vi "Message_Manager.vi"(6 "Log only on Err":bool, 7 "Action (Add)":T1, 8 "error in":errorcluster, 10 "New Entry":string, 11 "Log History Size (1000)":i32=1000) -> (0 "error out":errorcluster, 2 "Last Err":cluster{"code":i32, "source":string}, 3 "First Err (Latched)":cluster{"code":i32, "source":string}, 4 "Last Message":string="12/05/2020 06:01:50.239 PM -- hello world", 5 "Message Log":string="12/05/2020 06:01:50.239 PM -- hello world\r\n12/05/2020 06:01:50.238 PM -- hello world\r\n12/05/2020 06:01:50.237 PM -- hello world\r\n12/05/2020 06:01:50.237 PM -- hello world\r\n12/05/2020 06:01:50.236 PM -- hello world\r\n12/05/2020 06:01:50.235 PM -- hello world\r\n12/05/2020 06:01:50.234 PM -- hello world\r\n12/05/2020 06:01:50.234 PM -- hello world\r\n12/05/2020 06:01:50.233 PM -- hello world\r\n12/05/2020 06:01:50.232 PM -- hello world\r\n12/05/2020 06:01:50.231 PM -- hello world\r\n12/05/2020 06:01:50.231 PM -- hello world\r\n12/05/2020 06:01:50.230 PM -- hello world\r\n12/05/2020 06:01:50.227 PM -- hello world\r\n12/05/2020 06:01:50.227 PM -- hello world\r\n12/05/2020 06:01:50.226 PM -- hello world\r\n12/05/2020 06:01:50.225 PM -- hello world\r\n12/05/2020 06:01:50.224 PM -- hello world\r\n12/05/2020 06:01:50.224 PM -- hello world\r\n12/05/2020 06:01:50.223 PM -- hello world\r\n12/05/2020 06:01:50.222 PM -- hello world\r\n12/05/2020 06:01:50.221 PM -- hello world\r\n12/05/2020 06:01:50.221 PM -- hello world\r\n12/05/2020 06:01:50.220 PM -- hello world\r\n12/05/2020 06:01:50.219 PM -- hello world\r\n12/05/2020 06:01:50.218 PM -- hello world\r\n12/05/2020 06:01:50.218 PM -- hello world\r\n12/05/2020 06:01:50.217 PM -- hello world\r\n12/05/2020 06:01:50.216 PM -- hello world\r\n12/05/2020 06:01:50.215 PM -- hello world\r\n12/05/2020 06:01:50.215 PM -- hello world\r\n12/05/2020 06:01:50.215 PM -- hello world\r\n12/05/2020 06:01:50.213 PM -- hello world\r\n12/05/2020 06:01:50.211 PM -- hello world\r\n12/05/2020 06:01:50.211 PM -- hello world\r\n12/05/2020 06:01:50.210 PM -- hello world\r\n12/05/2020 06:01:50.209 PM -- hello world\r\n12/05/2020 06:01:50.208 PM -- hello world\r\n12/05/2020 06:01:50.208 PM -- hello world\r\n12/05/2020 06:01:50.207 PM -- hello world\r\n12/05/2020 06:01:50.206 PM -- hello world\r\n12/05/2020 06:01:50.205 PM -- hello world\r\n12/05/2020 06:01:50.205 PM -- hello world\r\n12/05/2020 06:01:50.204 PM -- hello world\r\n12/05/2020 06:01:50.203 PM -- hello world\r\n12/05/2020 06:01:50.203 PM -- hello world\r\n12/05/2020 06:01:50.202 PM -- hello world\r\n12/05/2020 06:01:50.201 PM -- hello world\r\n12/05/2020 06:01:50.200 PM -- hello world\r\n12/05/2020 06:01:50.200 PM -- hello world\r\n12/05/2020 06:01:50.199 PM -- hello world\r\n12/05/2020 06:01:50.198 PM -- hello world\r\n12/05/2020 06:01:50.196 PM -- hello world\r\n12/05/2020 06:01:50.195 PM -- hello world\r\n12/05/2020 06:01:50.194 PM -- hello world\r\n12/05/2020 06:01:50.193 PM -- hello world\r\n12/05/2020 06:01:50.193 PM -- hello world\r\n12/05/2020 06:01:50.192 PM -- hello world\r\n12/05/2020 06:01:50.191 PM -- hello world\r\n12/05/2020 06:01:50.191 PM -- hello world\r\n12/05/2020 06:01:50.190 PM -- hello world\r\n12/05/2020 06:01:50.189 PM -- hello world\r\n12/05/2020 06:01:50.188 PM -- hello world\r\n12/05/2020 06:01:50.188 PM -- hello world\r\n12/05/2020 06:01:50.187 PM -- hello world\r\n12/05/2020 06:01:50.186 PM -- hello world\r\n12/05/2020 06:01:50.186 PM -- hello world\r\n12/05/2020 06:01:50.185 PM -- hello world\r\n12/05/2020 06:01:50.184 PM -- hello world\r\n12/05/2020 06:01:50.183 PM -- hello world\r\n12/05/2020 06:01:50.182 PM -- hello world\r\n12/05/2020 06:01:50.180 PM -- hello world\r\n12/05/2020 06:01:50.179 PM -- hello world\r\n12/05/2020 06:01:50.179 PM -- hello world\r\n12/05/2020 06:01:50.178 PM -- hello world\r\n12/05/2020 06:01:50.177 PM -- hello world\r\n12/05/2020 06:01:50.176 PM -- hello world\r\n12/05/2020 06:01:50.175 PM -- hello world\r\n12/05/2020 06:01:50.175 PM -- hello world\r\n12/05/2020 06:01:50.174 PM -- hello world\r\n12/05/2020 06:01:50.173 PM -- hello world\r\n12/05/2020 06:01:50.173 PM -- hello world\r\n12/05/2020 06:01:50.173 PM -- hello world\r\n12/05/2020 06:01:50.172 PM -- hello world\r\n12/05/2020 06:01:50.171 PM -- hello world\r\n12/05/2020 06:01:50.171 PM -- hello world\r\n12/05/2020 06:01:50.170 PM -- hello world\r\n12/05/2020 06:01:50.169 PM -- hello world\r\n12/05/2020 06:01:50.168 PM -- hello world\r\n12/05/2020 06:01:50.167 PM -- hello world\r\n12/05/2020 06:01:50.166 PM -- hello world\r\n12/05/2020 06:01:50.166 PM -- hello world\r\n12/05/2020 06:01:50.165 PM -- hello world\r\n12/05/2020 06:01:50.164 PM -- hello world\r\n12/05/2020 06:01:50.164 PM -- hello world\r\n12/05/2020 06:01:50.163 PM -- hello world\r\n12/05/2020 06:01:50.161 PM -- hello world\r\n12/05/2020 06:01:50.160 PM -- hello world\r\n12/05/2020 06:01:50.159 PM -- hello world\r\n12/05/2020 06:01:50.159 PM -- hello world\r\n12/05/2020 06:01:50.158 PM -- hello world\r\n12/05/2020 06:01:50.157 PM -- hello world\r\n12/05/2020 06:01:50.156 PM -- hello world\r\n12/05/2020 06:01:50.156 PM -- hello world\r\n12/05/2020 06:01:50.155 PM -- hello world\r\n12/05/2020 06:01:50.154 PM -- hello world\r\n12/05/2020 06:01:50.153 PM -- hello world\r\n12/05/2020 06:01:50.153 PM -- hello world\r\n12/05/2020 06:01:50.152 PM -- hello world\r\n12/05/2020 06:01:50.151 PM -- hello world\r\n12/05/2020 06:01:50.150 PM -- hello world\r\n12/05/2020 06:01:50.148 PM -- hello world\r\n12/05/2020 06:01:50.147 PM -- hello world\r\n12/05/2020 06:01:50.147 PM -- hello world\r\n12/05/2020 06:01:50.146 PM -- hello world\r\n12/05/2020 06:01:50.145 PM -- hello world\r\n12/05/2020 06:01:50.144 PM -- hello world\r\n12/05/2020 06:01:50.143 PM -- hello world\r\n12/05/2020 06:01:50.142 PM -- hello world\r\n12/05/2020 06:01:50.142 PM -- hello world\r\n12/05/2020 06:01:50.141 PM -- hello world\r\n12/05/2020 06:01:50.140 PM -- hello world\r\n12/05/2020 06:01:50.139 PM -- hello world\r\n12/05/2020 06:01:50.138 PM -- hello world\r\n12/05/2020 06:01:50.137 PM -- hello world\r\n12/05/2020 06:01:50.137 PM -- hello world\r\n12/05/2020 06:01:50.136 PM -- hello world\r\n12/05/2020 06:01:50.135 PM -- hello world\r\n12/05/2020 06:01:50.133 PM -- hello world\r\n12/05/2020 06:01:50.133 PM -- hello world\r\n12/05/2020 06:01:50.132 PM -- hello world\r\n12/05/2020 06:01:50.131 PM -- hello world\r\n12/05/2020 06:01:50.130 PM -- hello world\r\n12/05/2020 06:01:50.130 PM -- hello world\r\n12/05/2020 06:01:50.130 PM -- hello world\r\n12/05/2020 06:01:50.129 PM -- hello world\r\n12/05/2020 06:01:50.128 PM -- hello world\r\n12/05/2020 06:01:50.127 PM -- hello world\r\n12/05/2020 06:01:50.127 PM -- hello world\r\n12/05/2020 06:01:50.126 PM -- hello world\r\n12/05/2020 06:01:50.125 PM -- hello world\r\n12/05/2020 06:01:50.124 PM -- hello world\r\n12/05/2020 06:01:50.124 PM -- hello world\r\n12/05/2020 06:01:50.123 PM -- hello world\r\n12/05/2020 06:01:50.122 PM -- hello world\r\n12/05/2020 06:01:50.121 PM -- hello world\r\n12/05/2020 06:01:50.121 PM -- hello world\r\n12/05/2020 06:01:50.120 PM -- hello world\r\n12/05/2020 06:01:50.119 PM -- hello world\r\n12/05/2020 06:01:50.118 PM -- hello world\r\n12/05/2020 06:01:50.117 PM -- hello world\r\n12/05/2020 06:01:50.117 PM -- hello world\r\n12/05/2020 06:01:50.116 PM -- hello world\r\n12/05/2020 06:01:50.115 PM -- hello world\r\n12/05/2020 06:01:50.114 PM -- hello world\r\n12/05/2020 06:01:50.114 PM -- hello world\r\n12/05/2020 06:01:50.113 PM -- hello world\r\n12/05/2020 06:01:50.112 PM -- hello world\r\n12/05/2020 06:01:50.111 PM -- hello world\r\n12/05/2020 06:01:50.111 PM -- hello world\r\n12/05/2020 06:01:50.110 PM -- hello world\r\n12/05/2020 06:01:50.109 PM -- hello world\r\n12/05/2020 06:01:50.108 PM -- hello world\r\n12/05/2020 06:01:50.108 PM -- hello world\r\n12/05/2020 06:01:50.107 PM -- hello world\r\n12/05/2020 06:01:50.106 PM -- hello world\r\n12/05/2020 06:01:50.105 PM -- hello world\r\n12/05/2020 06:01:50.105 PM -- hello world\r\n12/05/2020 06:01:50.102 PM -- hello world\r\n12/05/2020 06:01:50.102 PM -- hello world\r\n12/05/2020 06:01:50.101 PM -- hello world\r\n12/05/2020 06:01:50.100 PM -- hello world\r\n12/05/2020 06:01:50.099 PM -- hello world\r\n12/05/2020 06:01:50.099 PM -- hello world\r\n12/05/2020 06:01:50.098 PM -- hello world\r\n12/05/2020 06:01:50.097 PM -- hello world\r\n12/05/2020 06:01:50.096 PM -- hello world\r\n12/05/2020 06:01:50.096 PM -- hello world\r\n12/05/2020 06:01:50.095 PM -- hello world\r\n12/05/2020 06:01:50.094 PM -- hello world\r\n12/05/2020 06:01:50.093 PM -- hello world\r\n12/05/2020 06:01:50.092 PM -- hello world\r\n12/05/2020 06:01:50.091 PM -- hello world\r\n12/05/2020 06:01:50.091 PM -- hello world\r\n12/05/2020 06:01:50.090 PM -- hello world\r\n12/05/2020 06:01:50.090 PM -- hello world\r\n12/05/2020 06:01:50.090 PM -- hello world\r\n12/05/2020 06:01:50.089 PM -- hello world\r\n12/05/2020 06:01:50.086 PM -- hello world\r\n12/05/2020 06:01:50.086 PM -- hello world\r\n12/05/2020 06:01:50.085 PM -- hello world\r\n12/05/2020 06:01:50.084 PM -- hello world\r\n12/05/2020 06:01:50.083 PM -- hello world\r\n12/05/2020 06:01:50.083 PM -- hello world\r\n12/05/2020 06:01:50.082 PM -- hello world\r\n12/05/2020 06:01:50.081 PM -- hello world\r\n12/05/2020 06:01:50.080 PM -- hello world\r\n12/05/2020 06:01:50.079 PM -- hello world\r\n12/05/2020 06:01:50.077 PM -- hello world\r\n12/05/2020 06:01:50.075 PM -- hello world\r\n12/05/2020 06:01:50.073 PM -- hello world\r\n12/05/2020 06:01:50.073 PM -- hello world\r\n12/05/2020 06:01:50.072 PM -- hello world\r\n12/05/2020 06:01:50.071 PM -- hello world\r\n12/05/2020 06:01:50.070 PM -- hello world\r\n12/05/2020 06:01:50.070 PM -- hello world\r\n12/05/2020 06:01:50.069 PM -- hello world\r\n12/05/2020 06:01:50.068 PM -- hello world\r\n12/05/2020 06:01:50.067 PM -- hello world\r\n12/05/2020 06:01:50.066 PM -- hello world\r\n12/05/2020 06:01:50.066 PM -- hello world\r\n12/05/2020 06:01:50.065 PM -- hello world\r\n12/05/2020 06:01:50.064 PM -- hello world\r\n12/05/2020 06:01:50.064 PM -- hello world\r\n12/05/2020 06:01:50.063 PM -- hello world\r\n12/05/2020 06:01:50.062 PM -- hello world\r\n12/05/2020 06:01:50.061 PM -- hello world\r\n12/05/2020 06:01:50.060 PM -- hello world\r\n12/05/2020 06:01:50.059 PM -- hello world\r\n12/05/2020 06:01:50.058 PM -- hello world\r\n12/05/2020 06:01:50.056 PM -- hello world\r\n12/05/2020 06:01:50.053 PM -- hello world\r\n12/05/2020 06:01:50.051 PM -- hello world\r\n12/05/2020 06:01:50.049 PM -- hello world\r\n12/05/2020 06:01:50.048 PM -- hello world\r\n12/05/2020 06:01:50.046 PM -- hello world\r\n12/05/2020 06:01:50.042 PM -- hello world\r\n12/05/2020 06:01:50.039 PM -- hello world\r\n12/05/2020 06:01:50.038 PM -- hello world\r\n12/05/2020 06:01:50.037 PM -- hello world\r\n12/05/2020 06:01:50.037 PM -- hello world\r\n12/05/2020 06:01:50.036 PM -- hello world\r\n12/05/2020 06:01:50.035 PM -- hello world\r\n12/05/2020 06:01:50.034 PM -- hello world\r\n12/05/2020 06:01:50.033 PM -- hello world\r\n12/05/2020 06:01:50.033 PM -- hello world\r\n12/05/2020 06:01:50.032 PM -- hello world\r\n12/05/2020 06:01:50.031 PM -- hello world\r\n12/05/2020 06:01:50.031 PM -- hello world\r\n12/05/2020 06:01:50.030 PM -- hello world\r\n12/05/2020 06:01:50.029 PM -- hello world\r\n12/05/2020 06:01:50.028 PM -- hello world\r\n12/05/2020 06:01:50.026 PM -- hello world\r\n12/05/2020 06:01:50.023 PM -- hello world\r\n12/05/2020 06:01:50.023 PM -- hello world\r\n12/05/2020 06:01:50.022 PM -- hello world\r\n12/05/2020 06:01:50.021 PM -- hello world\r\n12/05/2020 06:01:50.020 PM -- hello world\r\n12/05/2020 06:01:50.020 PM -- hello world\r\n12/05/2020 06:01:50.019 PM -- hello world\r\n12/05/2020 06:01:50.018 PM -- hello world\r\n12/05/2020 06:01:50.017 PM -- hello world\r\n12/05/2020 06:01:50.016 PM -- hello world\r\n12/05/2020 06:01:50.015 PM -- hello world\r\n12/05/2020 06:01:50.014 PM -- hello world\r\n12/05/2020 06:01:50.013 PM -- hello world\r\n12/05/2020 06:01:50.012 PM -- hello world\r\n12/05/2020 06:01:50.012 PM -- hello world\r\n12/05/2020 06:01:50.011 PM -- hello world\r\n12/05/2020 06:01:50.010 PM -- hello world\r\n12/05/2020 06:01:50.009 PM -- hello world\r\n12/05/2020 06:01:50.009 PM -- hello world\r\n12/05/2020 06:01:50.007 PM -- hello world\r\n12/05/2020 06:01:50.006 PM -- hello world\r\n12/05/2020 06:01:50.006 PM -- hello world\r\n12/05/2020 06:01:50.006 PM -- hello world\r\n12/05/2020 06:01:50.005 PM -- hello world\r\n12/05/2020 06:01:50.004 PM -- hello world\r\n12/05/2020 06:01:50.004 PM -- hello world\r\n12/05/2020 06:01:50.003 PM -- hello world\r\n12/05/2020 06:01:50.002 PM -- hello world\r\n12/05/2020 06:01:50.001 PM -- hello world\r\n12/05/2020 06:01:50.001 PM -- hello world\r\n12/05/2020 06:01:50.000 PM -- hello world\r\n12/05/2020 06:01:49.999 PM -- hello world\r\n12/05/2020 06:01:49.999 PM -- hello world\r\n12/05/2020 06:01:49.998 PM -- hello world\r\n12/05/2020 06:01:49.997 PM -- hello world\r\n12/05/2020 06:01:49.994 PM -- hello world\r\n12/05/2020 06:01:49.993 PM -- hello world\r\n12/05/2020 06:01:49.992 PM -- hello world\r\n12/05/2020 06:01:49.991 PM -- hello world\r\n12/05/2020 06:01:49.991 PM -- hello world\r\n12/05/2020 06:01:49.990 PM -- hello world\r\n12/05/2020 06:01:49.989 PM -- hello world\r\n12/05/2020 06:01:49.988 PM -- hello world\r\n12/05/2020 06:01:49.988 PM -- hello world\r\n12/05/2020 06:01:49.987 PM -- hello world\r\n12/05/2020 06:01:49.986 PM -- hello world\r\n12/05/2020 06:01:49.986 PM -- hello world\r\n12/05/2020 06:01:49.985 PM -- hello world\r\n12/05/2020 06:01:49.984 PM -- hello world\r\n12/05/2020 06:01:49.983 PM -- hello world\r\n12/05/2020 06:01:49.982 PM -- hello world\r\n12/05/2020 06:01:49.982 PM -- hello world\r\n12/05/2020 06:01:49.981 PM -- hello world\r\n12/05/2020 06:01:49.980 PM -- hello world\r\n12/05/2020 06:01:49.980 PM -- hello world\r\n12/05/2020 06:01:49.979 PM -- hello world\r\n12/05/2020 06:01:49.976 PM -- hello world\r\n12/05/2020 06:01:49.976 PM -- hello world\r\n12/05/2020 06:01:49.975 PM -- hello world\r\n12/05/2020 06:01:49.974 PM -- hello world\r\n12/05/2020 06:01:49.973 PM -- hello world\r\n12/05/2020 06:01:49.973 PM -- hello world\r\n12/05/2020 06:01:49.972 PM -- hello world\r\n12/05/2020 06:01:49.971 PM -- hello world\r\n12/05/2020 06:01:49.971 PM -- hello world\r\n12/05/2020 06:01:49.970 PM -- hello world\r\n12/05/2020 06:01:49.969 PM -- hello world\r\n12/05/2020 06:01:49.968 PM -- hello world\r\n12/05/2020 06:01:49.968 PM -- hello world\r\n12/05/2020 06:01:49.967 PM -- hello world\r\n12/05/2020 06:01:49.966 PM -- hello world\r\n12/05/2020 06:01:49.965 PM -- hello world\r\n12/05/2020 06:01:49.965 PM -- hello world\r\n12/05/2020 06:01:49.965 PM -- hello world\r\n12/05/2020 06:01:49.963 PM -- hello world\r\n12/05/2020 06:01:49.961 PM -- hello world\r\n12/05/2020 06:01:49.960 PM -- hello world\r\n12/05/2020 06:01:49.960 PM -- hello world\r\n12/05/2020 06:01:49.959 PM -- hello world\r\n12/05/2020 06:01:49.958 PM -- hello world\r\n12/05/2020 06:01:49.957 PM -- hello world\r\n12/05/2020 06:01:49.957 PM -- hello world\r\n12/05/2020 06:01:49.956 PM -- hello world\r\n12/05/2020 06:01:49.955 PM -- hello world\r\n12/05/2020 06:01:49.955 PM -- hello world\r\n12/05/2020 06:01:49.954 PM -- hello world\r\n12/05/2020 06:01:49.953 PM -- hello world\r\n12/05/2020 06:01:49.952 PM -- hello world\r\n12/05/2020 06:01:49.952 PM -- hello world\r\n12/05/2020 06:01:49.951 PM -- hello world\r\n12/05/2020 06:01:49.950 PM -- hello world\r\n12/05/2020 06:01:49.949 PM -- hello world\r\n12/05/2020 06:01:49.948 PM -- hello world\r\n12/05/2020 06:01:49.948 PM -- hello world\r\n12/05/2020 06:01:49.945 PM -- hello world\r\n12/05/2020 06:01:49.944 PM -- hello world\r\n12/05/2020 06:01:49.944 PM -- hello world\r\n12/05/2020 06:01:49.942 PM -- hello world\r\n12/05/2020 06:01:49.941 PM -- hello world\r\n12/05/2020 06:01:49.940 PM -- hello world\r\n12/05/2020 06:01:49.940 PM -- hello world\r\n12/05/2020 06:01:49.939 PM -- hello world\r\n12/05/2020 06:01:49.938 PM -- hello world\r\n12/05/2020 06:01:49.938 PM -- hello world\r\n12/05/2020 06:01:49.937 PM -- hello world\r\n12/05/2020 06:01:49.936 PM -- hello world\r\n12/05/2020 06:01:49.935 PM -- hello world\r\n12/05/2020 06:01:49.935 PM -- hello world\r\n12/05/2020 06:01:49.933 PM -- hello world\r\n12/05/2020 06:01:49.932 PM -- hello world\r\n12/05/2020 06:01:49.930 PM -- hello world\r\n12/05/2020 06:01:49.929 PM -- hello world\r\n12/05/2020 06:01:49.928 PM -- hello world\r\n12/05/2020 06:01:49.928 PM -- hello world\r\n12/05/2020 06:01:49.927 PM -- hello world\r\n12/05/2020 06:01:49.926 PM -- hello world\r\n12/05/2020 06:01:49.925 PM -- hello world\r\n12/05/2020 06:01:49.925 PM -- hello world\r\n12/05/2020 06:01:49.924 PM -- hello world\r\n12/05/2020 06:01:49.923 PM -- hello world\r\n12/05/2020 06:01:49.923 PM -- hello world\r\n12/05/2020 06:01:49.923 PM -- hello world\r\n12/05/2020 06:01:49.922 PM -- hello world\r\n12/05/2020 06:01:49.921 PM -- hello world\r\n12/05/2020 06:01:49.921 PM -- hello world\r\n12/05/2020 06:01:49.920 PM -- hello world\r\n12/05/2020 06:01:49.919 PM -- hello world\r\n12/05/2020 06:01:49.919 PM -- hello world\r\n12/05/2020 06:01:49.918 PM -- hello world\r\n12/05/2020 06:01:49.917 PM -- hello world\r\n12/05/2020 06:01:49.916 PM -- hello world\r\n12/05/2020 06:01:49.914 PM -- hello world\r\n12/05/2020 06:01:49.914 PM -- hello world\r\n12/05/2020 06:01:49.913 PM -- hello world\r\n12/05/2020 06:01:49.912 PM -- hello world\r\n12/05/2020 06:01:49.912 PM -- hello world\r\n12/05/2020 06:01:49.911 PM -- hello world\r\n12/05/2020 06:01:49.910 PM -- hello world\r\n12/05/2020 06:01:49.909 PM -- hello world\r\n12/05/2020 06:01:49.908 PM -- hello world\r\n12/05/2020 06:01:49.908 PM -- hello world\r\n12/05/2020 06:01:49.907 PM -- hello world\r\n12/05/2020 06:01:49.906 PM -- hello world\r\n12/05/2020 06:01:49.905 PM -- hello world\r\n12/05/2020 06:01:49.905 PM -- hello world\r\n12/05/2020 06:01:49.904 PM -- hello world\r\n12/05/2020 06:01:49.903 PM -- hello world\r\n12/05/2020 06:01:49.903 PM -- hello world\r\n12/05/2020 06:01:49.899 PM -- hello world\r\n12/05/2020 06:01:49.899 PM -- hello world\r\n12/05/2020 06:01:49.898 PM -- hello world\r\n12/05/2020 06:01:49.897 PM -- hello world\r\n12/05/2020 06:01:49.896 PM -- hello world\r\n12/05/2020 06:01:49.896 PM -- hello world\r\n12/05/2020 06:01:49.895 PM -- hello world\r\n12/05/2020 06:01:49.894 PM -- hello world\r\n12/05/2020 06:01:49.893 PM -- hello world\r\n12/05/2020 06:01:49.892 PM -- hello world\r\n12/05/2020 06:01:49.892 PM -- hello world\r\n12/05/2020 06:01:49.891 PM -- hello world\r\n12/05/2020 06:01:49.890 PM -- hello world\r\n12/05/2020 06:01:49.889 PM -- hello world\r\n12/05/2020 06:01:49.889 PM -- hello world\r\n12/05/2020 06:01:49.888 PM -- hello world\r\n12/05/2020 06:01:49.887 PM -- hello world\r\n12/05/2020 06:01:49.886 PM -- hello world\r\n12/05/2020 06:01:49.885 PM -- hello world\r\n12/05/2020 06:01:49.884 PM -- hello world\r\n12/05/2020 06:01:49.883 PM -- hello world\r\n12/05/2020 06:01:49.883 PM -- hello world\r\n12/05/2020 06:01:49.882 PM -- hello world\r\n12/05/2020 06:01:49.881 PM -- hello world\r\n12/05/2020 06:01:49.881 PM -- hello world\r\n12/05/2020 06:01:49.881 PM -- hello world\r\n12/05/2020 06:01:49.880 PM -- hello world\r\n12/05/2020 06:01:49.879 PM -- hello world\r\n12/05/2020 06:01:49.878 PM -- hello world\r\n12/05/2020 06:01:49.877 PM -- hello world\r\n12/05/2020 06:01:49.876 PM -- hello world\r\n12/05/2020 06:01:49.875 PM -- hello world\r\n12/05/2020 06:01:49.874 PM -- hello world\r\n12/05/2020 06:01:49.874 PM -- hello world\r\n12/05/2020 06:01:49.873 PM -- hello world\r\n12/05/2020 06:01:49.872 PM -- hello world\r\n12/05/2020 06:01:49.871 PM -- hello world\r\n12/05/2020 06:01:49.871 PM -- hello world\r\n12/05/2020 06:01:49.870 PM -- hello world\r\n12/05/2020 06:01:49.869 PM -- hello world\r\n12/05/2020 06:01:49.869 PM -- hello world\r\n12/05/2020 06:01:49.867 PM -- hello world\r\n12/05/2020 06:01:49.867 PM -- hello world\r\n12/05/2020 06:01:49.866 PM -- hello world\r\n12/05/2020 06:01:49.865 PM -- hello world\r\n12/05/2020 06:01:49.865 PM -- hello world\r\n12/05/2020 06:01:49.864 PM -- hello world\r\n12/05/2020 06:01:49.863 PM -- hello world\r\n12/05/2020 06:01:49.863 PM -- hello world\r\n12/05/2020 06:01:49.862 PM -- hello world\r\n12/05/2020 06:01:49.861 PM -- hello world\r\n12/05/2020 06:01:49.860 PM -- hello world\r\n12/05/2020 06:01:49.860 PM -- hello world\r\n12/05/2020 06:01:49.859 PM -- hello world\r\n12/05/2020 06:01:49.858 PM -- hello world\r\n12/05/2020 06:01:49.857 PM -- hello world\r\n12/05/2020 06:01:49.856 PM -- hello world\r\n12/05/2020 06:01:49.855 PM -- hello world\r\n12/05/2020 06:01:49.855 PM -- hello world\r\n12/05/2020 06:01:49.851 PM -- hello world\r\n12/05/2020 06:01:49.851 PM -- hello world\r\n12/05/2020 06:01:49.850 PM -- hello world\r\n12/05/2020 06:01:49.849 PM -- hello world\r\n12/05/2020 06:01:49.849 PM -- hello world\r\n12/05/2020 06:01:49.848 PM -- hello world\r\n12/05/2020 06:01:49.847 PM -- hello world\r\n12/05/2020 06:01:49.846 PM -- hello world\r\n12/05/2020 06:01:49.845 PM -- hello world\r\n12/05/2020 06:01:49.844 PM -- hello world\r\n12/05/2020 06:01:49.844 PM -- hello world\r\n12/05/2020 06:01:49.843 PM -- hello world\r\n12/05/2020 06:01:49.842 PM -- hello world\r\n12/05/2020 06:01:49.842 PM -- hello world\r\n12/05/2020 06:01:49.840 PM -- hello world\r\n12/05/2020 06:01:49.840 PM -- hello world\r\n12/05/2020 06:01:49.839 PM -- hello world\r\n12/05/2020 06:01:49.836 PM -- hello world\r\n12/05/2020 06:01:49.836 PM -- hello world\r\n12/05/2020 06:01:49.834 PM -- hello world\r\n12/05/2020 06:01:49.833 PM -- hello world\r\n12/05/2020 06:01:49.833 PM -- hello world\r\n12/05/2020 06:01:49.832 PM -- hello world\r\n12/05/2020 06:01:49.831 PM -- hello world\r\n12/05/2020 06:01:49.830 PM -- hello world\r\n12/05/2020 06:01:49.829 PM -- hello world\r\n12/05/2020 06:01:49.828 PM -- hello world\r\n12/05/2020 06:01:49.828 PM -- hello world\r\n12/05/2020 06:01:49.827 PM -- hello world\r\n12/05/2020 06:01:49.826 PM -- hello world\r\n12/05/2020 06:01:49.825 PM -- hello world\r\n12/05/2020 06:01:49.824 PM -- hello world\r\n12/05/2020 06:01:49.824 PM -- hello world\r\n12/05/2020 06:01:49.823 PM -- hello world\r\n12/05/2020 06:01:49.820 PM -- hello world\r\n12/05/2020 06:01:49.819 PM -- hello world\r\n12/05/2020 06:01:49.818 PM -- hello world\r\n12/05/2020 06:01:49.818 PM -- hello world\r\n12/05/2020 06:01:49.817 PM -- hello world\r\n12/05/2020 06:01:49.816 PM -- hello world\r\n12/05/2020 06:01:49.815 PM -- hello world\r\n12/05/2020 06:01:49.814 PM -- hello world\r\n12/05/2020 06:01:49.813 PM -- hello world\r\n12/05/2020 06:01:49.812 PM -- hello world\r\n12/05/2020 06:01:49.811 PM -- hello world\r\n12/05/2020 06:01:49.810 PM -- hello world\r\n12/05/2020 06:01:49.809 PM -- hello world\r\n12/05/2020 06:01:49.808 PM -- hello world\r\n12/05/2020 06:01:49.807 PM -- hello world\r\n12/05/2020 06:01:49.807 PM -- hello world\r\n12/05/2020 06:01:49.805 PM -- hello world\r\n12/05/2020 06:01:49.805 PM -- hello world\r\n12/05/2020 06:01:49.804 PM -- hello world\r\n12/05/2020 06:01:49.803 PM -- hello world\r\n12/05/2020 06:01:49.803 PM -- hello world\r\n12/05/2020 06:01:49.801 PM -- hello world\r\n12/05/2020 06:01:49.800 PM -- hello world\r\n12/05/2020 06:01:49.800 PM -- hello world\r\n12/05/2020 06:01:49.799 PM -- hello world\r\n12/05/2020 06:01:49.798 PM -- hello world\r\n12/05/2020 06:01:49.798 PM -- hello world\r\n12/05/2020 06:01:49.797 PM -- hello world\r\n12/05/2020 06:01:49.795 PM -- hello world\r\n12/05/2020 06:01:49.793 PM -- hello world\r\n12/05/2020 06:01:49.792 PM -- hello world\r\n12/05/2020 06:01:49.791 PM -- hello world\r\n12/05/2020 06:01:49.790 PM -- hello world\r\n12/05/2020 06:01:49.790 PM -- hello world\r\n12/05/2020 06:01:49.789 PM -- hello world\r\n12/05/2020 06:01:49.788 PM -- hello world\r\n12/05/2020 06:01:49.788 PM -- hello world\r\n12/05/2020 06:01:49.787 PM -- hello world\r\n12/05/2020 06:01:49.786 PM -- hello world\r\n12/05/2020 06:01:49.785 PM -- hello world\r\n12/05/2020 06:01:49.784 PM -- hello world\r\n12/05/2020 06:01:49.783 PM -- hello world\r\n12/05/2020 06:01:49.782 PM -- hello world\r\n12/05/2020 06:01:49.781 PM -- hello world\r\n12/05/2020 06:01:49.780 PM -- hello world\r\n12/05/2020 06:01:49.778 PM -- hello world\r\n12/05/2020 06:01:49.777 PM -- hello world\r\n12/05/2020 06:01:49.776 PM -- hello world\r\n12/05/2020 06:01:49.775 PM -- hello world\r\n12/05/2020 06:01:49.773 PM -- hello world\r\n12/05/2020 06:01:49.772 PM -- hello world\r\n12/05/2020 06:01:49.771 PM -- hello world\r\n12/05/2020 06:01:49.771 PM -- hello world\r\n12/05/2020 06:01:49.770 PM -- hello world\r\n12/05/2020 06:01:49.769 PM -- hello world\r\n12/05/2020 06:01:49.767 PM -- hello world\r\n12/05/2020 06:01:49.767 PM -- hello world\r\n12/05/2020 06:01:49.766 PM -- hello world\r\n12/05/2020 06:01:49.765 PM -- hello world\r\n12/05/2020 06:01:49.764 PM -- hello world\r\n12/05/2020 06:01:49.762 PM -- hello world\r\n12/05/2020 06:01:49.761 PM -- hello world\r\n12/05/2020 06:01:49.759 PM -- hello world\r\n12/05/2020 06:01:49.758 PM -- hello world\r\n12/05/2020 06:01:49.757 PM -- hello world\r\n12/05/2020 06:01:49.756 PM -- hello world\r\n12/05/2020 06:01:49.756 PM -- hello world\r\n12/05/2020 06:01:49.755 PM -- hello world\r\n12/05/2020 06:01:49.754 PM -- hello world\r\n12/05/2020 06:01:49.753 PM -- hello world\r\n12/05/2020 06:01:49.752 PM -- hello world\r\n12/05/2020 06:01:49.752 PM -- hello world\r\n12/05/2020 06:01:49.751 PM -- hello world\r\n12/05/2020 06:01:49.750 PM -- hello world\r\n12/05/2020 06:01:49.750 PM -- hello world\r\n12/05/2020 06:01:49.749 PM -- hello world\r\n12/05/2020 06:01:49.748 PM -- hello world\r\n12/05/2020 06:01:49.747 PM -- hello world\r\n12/05/2020 06:01:49.747 PM -- hello world\r\n12/05/2020 06:01:49.746 PM -- hello world\r\n12/05/2020 06:01:49.745 PM -- hello world\r\n12/05/2020 06:01:49.745 PM -- hello world\r\n12/05/2020 06:01:49.744 PM -- hello world\r\n12/05/2020 06:01:49.742 PM -- hello world\r\n12/05/2020 06:01:49.742 PM -- hello world\r\n12/05/2020 06:01:49.741 PM -- hello world\r\n12/05/2020 06:01:49.740 PM -- hello world\r\n12/05/2020 06:01:49.739 PM -- hello world\r\n12/05/2020 06:01:49.739 PM -- hello world\r\n12/05/2020 06:01:49.738 PM -- hello world\r\n12/05/2020 06:01:49.737 PM -- hello world\r\n12/05/2020 06:01:49.736 PM -- hello world\r\n12/05/2020 06:01:49.736 PM -- hello world\r\n12/05/2020 06:01:49.735 PM -- hello world\r\n12/05/2020 06:01:49.734 PM -- hello world\r\n12/05/2020 06:01:49.733 PM -- hello world\r\n12/05/2020 06:01:49.733 PM -- hello world\r\n12/05/2020 06:01:49.732 PM -- hello world\r\n12/05/2020 06:01:49.731 PM -- hello world\r\n12/05/2020 06:01:49.730 PM -- hello world\r\n12/05/2020 06:01:49.729 PM -- hello world\r\n12/05/2020 06:01:49.727 PM -- hello world\r\n12/05/2020 06:01:49.726 PM -- hello world\r\n12/05/2020 06:01:49.726 PM -- hello world\r\n12/05/2020 06:01:49.725 PM -- hello world\r\n12/05/2020 06:01:49.724 PM -- hello world\r\n12/05/2020 06:01:49.724 PM -- hello world\r\n12/05/2020 06:01:49.723 PM -- hello world\r\n12/05/2020 06:01:49.722 PM -- hello world\r\n12/05/2020 06:01:49.721 PM -- hello world\r\n12/05/2020 06:01:49.721 PM -- hello world\r\n12/05/2020 06:01:49.720 PM -- hello world\r\n12/05/2020 06:01:49.719 PM -- hello world\r\n12/05/2020 06:01:49.719 PM -- hello world\r\n12/05/2020 06:01:49.718 PM -- hello world\r\n12/05/2020 06:01:49.717 PM -- hello world\r\n12/05/2020 06:01:49.716 PM -- hello world\r\n12/05/2020 06:01:49.716 PM -- hello world\r\n12/05/2020 06:01:49.715 PM -- hello world\r\n12/05/2020 06:01:49.715 PM -- hello world\r\n12/05/2020 06:01:49.715 PM -- hello world\r\n12/05/2020 06:01:49.714 PM -- hello world\r\n12/05/2020 06:01:49.713 PM -- hello world\r\n12/05/2020 06:01:49.712 PM -- hello world\r\n12/05/2020 06:01:49.711 PM -- hello world\r\n12/05/2020 06:01:49.710 PM -- hello world\r\n12/05/2020 06:01:49.709 PM -- hello world\r\n12/05/2020 06:01:49.709 PM -- hello world\r\n12/05/2020 06:01:49.708 PM -- hello world\r\n12/05/2020 06:01:49.707 PM -- hello world\r\n12/05/2020 06:01:49.707 PM -- hello world\r\n12/05/2020 06:01:49.706 PM -- hello world\r\n12/05/2020 06:01:49.705 PM -- hello world\r\n12/05/2020 06:01:49.704 PM -- hello world\r\n12/05/2020 06:01:49.704 PM -- hello world\r\n12/05/2020 06:01:49.703 PM -- hello world\r\n12/05/2020 06:01:49.702 PM -- hello world\r\n12/05/2020 06:01:49.701 PM -- hello world\r\n12/05/2020 06:01:49.701 PM -- hello world\r\n12/05/2020 06:01:49.700 PM -- hello world\r\n12/05/2020 06:01:49.699 PM -- hello world\r\n12/05/2020 06:01:49.699 PM -- hello world\r\n12/05/2020 06:01:49.698 PM -- hello world\r\n12/05/2020 06:01:49.696 PM -- hello world\r\n12/05/2020 06:01:49.695 PM -- hello world\r\n12/05/2020 06:01:49.694 PM -- hello world\r\n12/05/2020 06:01:49.693 PM -- hello world\r\n12/05/2020 06:01:49.692 PM -- hello world\r\n12/05/2020 06:01:49.692 PM -- hello world\r\n12/05/2020 06:01:49.691 PM -- hello world\r\n12/05/2020 06:01:49.690 PM -- hello world\r\n12/05/2020 06:01:49.689 PM -- hello world\r\n12/05/2020 06:01:49.689 PM -- hello world\r\n12/05/2020 06:01:49.688 PM -- hello world\r\n12/05/2020 06:01:49.687 PM -- hello world\r\n12/05/2020 06:01:49.686 PM -- hello world\r\n12/05/2020 06:01:49.685 PM -- hello world\r\n12/05/2020 06:01:49.684 PM -- hello world\r\n12/05/2020 06:01:49.684 PM -- hello world\r\n12/05/2020 06:01:49.683 PM -- hello world\r\n12/05/2020 06:01:49.682 PM -- hello world\r\n12/05/2020 06:01:49.680 PM -- hello world\r\n12/05/2020 06:01:49.679 PM -- hello world\r\n12/05/2020 06:01:49.679 PM -- hello world\r\n12/05/2020 06:01:49.678 PM -- hello world\r\n12/05/2020 06:01:49.677 PM -- hello world\r\n12/05/2020 06:01:49.677 PM -- hello world\r\n12/05/2020 06:01:49.676 PM -- hello world\r\n12/05/2020 06:01:49.675 PM -- hello world\r\n12/05/2020 06:01:49.674 PM -- hello world\r\n12/05/2020 06:01:49.674 PM -- hello world\r\n12/05/2020 06:01:49.673 PM -- hello world\r\n12/05/2020 06:01:49.673 PM -- hello world\r\n12/05/2020 06:01:49.673 PM -- hello world\r\n12/05/2020 06:01:49.672 PM -- hello world\r\n12/05/2020 06:01:49.671 PM -- hello world\r\n12/05/2020 06:01:49.669 PM -- hello world\r\n12/05/2020 06:01:49.668 PM -- hello world\r\n12/05/2020 06:01:49.667 PM -- hello world\r\n12/05/2020 06:01:49.667 PM -- hello world\r\n12/05/2020 06:01:49.666 PM -- hello world\r\n12/05/2020 06:01:49.665 PM -- hello world\r\n12/05/2020 06:01:49.664 PM -- hello world\r\n12/05/2020 06:01:49.664 PM -- hello world\r\n12/05/2020 06:01:49.663 PM -- hello world\r\n12/05/2020 06:01:49.662 PM -- hello world\r\n12/05/2020 06:01:49.661 PM -- hello world\r\n12/05/2020 06:01:49.661 PM -- hello world\r\n12/05/2020 06:01:49.660 PM -- hello world\r\n12/05/2020 06:01:49.659 PM -- hello world\r\n12/05/2020 06:01:49.659 PM -- hello world\r\n12/05/2020 06:01:49.657 PM -- hello world\r\n12/05/2020 06:01:49.657 PM -- hello world\r\n12/05/2020 06:01:49.656 PM -- hello world\r\n12/05/2020 06:01:49.655 PM -- hello world\r\n12/05/2020 06:01:49.654 PM -- hello world\r\n12/05/2020 06:01:49.654 PM -- hello world\r\n12/05/2020 06:01:49.653 PM -- hello world\r\n12/05/2020 06:01:49.652 PM -- hello world\r\n12/05/2020 06:01:49.652 PM -- hello world\r\n12/05/2020 06:01:49.651 PM -- hello world\r\n12/05/2020 06:01:49.648 PM -- hello world\r\n12/05/2020 06:01:49.648 PM -- hello world\r\n12/05/2020 06:01:49.647 PM -- hello world\r\n12/05/2020 06:01:49.646 PM -- hello world\r\n12/05/2020 06:01:49.645 PM -- hello world\r\n12/05/2020 06:01:49.645 PM -- hello world\r\n12/05/2020 06:01:49.644 PM -- hello world\r\n12/05/2020 06:01:49.643 PM -- hello world\r\n12/05/2020 06:01:49.643 PM -- hello world\r\n12/05/2020 06:01:49.642 PM -- hello world\r\n12/05/2020 06:01:49.641 PM -- hello world\r\n12/05/2020 06:01:49.639 PM -- hello world\r\n12/05/2020 06:01:49.638 PM -- hello world\r\n12/05/2020 06:01:49.637 PM -- hello world\r\n12/05/2020 06:01:49.637 PM -- hello world\r\n12/05/2020 06:01:49.636 PM -- hello world\r\n12/05/2020 06:01:49.635 PM -- hello world\r\n12/05/2020 06:01:49.635 PM -- hello world\r\n12/05/2020 06:01:49.634 PM -- hello world\r\n12/05/2020 06:01:49.632 PM -- hello world\r\n12/05/2020 06:01:49.632 PM -- hello world\r\n12/05/2020 06:01:49.632 PM -- hello world\r\n12/05/2020 06:01:49.631 PM -- hello world\r\n12/05/2020 06:01:49.630 PM -- hello world\r\n12/05/2020 06:01:49.630 PM -- hello world\r\n12/05/2020 06:01:49.629 PM -- hello world\r\n12/05/2020 06:01:49.628 PM -- hello world\r\n12/05/2020 06:01:49.627 PM -- hello world\r\n12/05/2020 06:01:49.627 PM -- hello world\r\n12/05/2020 06:01:49.626 PM -- hello world\r\n12/05/2020 06:01:49.625 PM -- hello world\r\n12/05/2020 06:01:49.624 PM -- hello world\r\n12/05/2020 06:01:49.624 PM -- hello world\r\n12/05/2020 06:01:49.623 PM -- hello world\r\n12/05/2020 06:01:49.622 PM -- hello world\r\n12/05/2020 06:01:49.622 PM -- hello world\r\n12/05/2020 06:01:49.621 PM -- hello world\r\n12/05/2020 06:01:49.620 PM -- hello world\r\n12/05/2020 06:01:49.618 PM -- hello world\r\n12/05/2020 06:01:49.618 PM -- hello world\r\n12/05/2020 06:01:49.617 PM -- hello world\r\n12/05/2020 06:01:49.616 PM -- hello world\r\n12/05/2020 06:01:49.615 PM -- hello world\r\n12/05/2020 06:01:49.615 PM -- hello world\r\n12/05/2020 06:01:49.614 PM -- hello world\r\n12/05/2020 06:01:49.613 PM -- hello world\r\n12/05/2020 06:01:49.612 PM -- hello world\r\n12/05/2020 06:01:49.611 PM -- hello world\r\n12/05/2020 06:01:49.611 PM -- hello world\r\n12/05/2020 06:01:49.610 PM -- hello world\r\n12/05/2020 06:01:49.609 PM -- hello world\r\n12/05/2020 06:01:49.609 PM -- hello world\r\n12/05/2020 06:01:49.608 PM -- hello world\r\n12/05/2020 06:01:49.607 PM -- hello world\r\n12/05/2020 06:01:49.606 PM -- hello world\r\n12/05/2020 06:01:49.606 PM -- hello world\r\n12/05/2020 06:01:49.605 PM -- hello world\r\n12/05/2020 06:01:49.604 PM -- hello world\r\n12/05/2020 06:01:49.603 PM -- hello world\r\n12/05/2020 06:01:49.601 PM -- hello world\r\n12/05/2020 06:01:49.600 PM -- hello world\r\n12/05/2020 06:01:49.600 PM -- hello world\r\n12/05/2020 06:01:49.599 PM -- hello world\r\n12/05/2020 06:01:49.598 PM -- hello world\r\n12/05/2020 06:01:49.598 PM -- hello world\r\n12/05/2020 06:01:49.597 PM -- hello world\r\n12/05/2020 06:01:49.596 PM -- hello world\r\n12/05/2020 06:01:49.595 PM -- hello world\r\n12/05/2020 06:01:49.594 PM -- hello world\r\n12/05/2020 06:01:49.594 PM -- hello world\r\n12/05/2020 06:01:49.593 PM -- hello world\r\n12/05/2020 06:01:49.592 PM -- hello world\r\n12/05/2020 06:01:49.591 PM -- hello world\r\n12/05/2020 06:01:49.590 PM -- hello world\r\n12/05/2020 06:01:49.590 PM -- hello world\r\n12/05/2020 06:01:49.590 PM -- hello world\r\n12/05/2020 06:01:49.588 PM -- hello world\r\n12/05/2020 06:01:49.586 PM -- hello world\r\n12/05/2020 06:01:49.586 PM -- hello world\r\n12/05/2020 06:01:49.585 PM -- hello world\r\n12/05/2020 06:01:49.584 PM -- hello world\r\n12/05/2020 06:01:49.583 PM -- hello world\r\n12/05/2020 06:01:49.582 PM -- hello world\r\n12/05/2020 06:01:49.582 PM -- hello world\r\n12/05/2020 06:01:49.581 PM -- hello world\r\n12/05/2020 06:01:49.580 PM -- hello world\r\n12/05/2020 06:01:49.580 PM -- hello world\r\n12/05/2020 06:01:49.579 PM -- hello world\r\n12/05/2020 06:01:49.578 PM -- hello world\r\n12/05/2020 06:01:49.577 PM -- hello world\r\n12/05/2020 06:01:49.576 PM -- hello world\r\n12/05/2020 06:01:49.575 PM -- hello world\r\n12/05/2020 06:01:49.574 PM -- hello world\r\n12/05/2020 06:01:49.571 PM -- hello world\r\n12/05/2020 06:01:49.571 PM -- hello world\r\n12/05/2020 06:01:49.570 PM -- hello world\r\n12/05/2020 06:01:49.569 PM -- hello world\r\n12/05/2020 06:01:49.568 PM -- hello world\r\n12/05/2020 06:01:49.568 PM -- hello world\r\n12/05/2020 06:01:49.566 PM -- hello world\r\n12/05/2020 06:01:49.565 PM -- hello world\r\n12/05/2020 06:01:49.564 PM -- hello world\r\n12/05/2020 06:01:49.563 PM -- hello world\r\n12/05/2020 06:01:49.562 PM -- hello world\r\n12/05/2020 06:01:49.561 PM -- hello world\r\n12/05/2020 06:01:49.560 PM -- hello world\r\n12/05/2020 06:01:49.560 PM -- hello world\r\n12/05/2020 06:01:49.559 PM -- hello world\r\n12/05/2020 06:01:49.558 PM -- hello world\r\n12/05/2020 06:01:49.557 PM -- hello world\r\n12/05/2020 06:01:49.555 PM -- hello world\r\n12/05/2020 06:01:49.555 PM -- hello world\r\n12/05/2020 06:01:49.554 PM -- hello world\r\n12/05/2020 06:01:49.553 PM -- hello world\r\n12/05/2020 06:01:49.552 PM -- hello world\r\n12/05/2020 06:01:49.552 PM -- hello world\r\n12/05/2020 06:01:49.551 PM -- hello world\r\n12/05/2020 06:01:49.550 PM -- hello world\r\n12/05/2020 06:01:49.549 PM -- hello world\r\n12/05/2020 06:01:49.549 PM -- hello world\r\n12/05/2020 06:01:49.549 PM -- hello world\r\n12/05/2020 06:01:49.548 PM -- hello world\r\n12/05/2020 06:01:49.547 PM -- hello world\r\n12/05/2020 06:01:49.547 PM -- hello world\r\n12/05/2020 06:01:49.546 PM -- hello world\r\n12/05/2020 06:01:49.545 PM -- hello world\r\n12/05/2020 06:01:49.544 PM -- hello world\r\n12/05/2020 06:01:49.543 PM -- hello world\r\n12/05/2020 06:01:49.541 PM -- hello world\r\n12/05/2020 06:01:49.539 PM -- hello world\r\n12/05/2020 06:01:49.539 PM -- hello world\r\n12/05/2020 06:01:49.538 PM -- hello world\r\n12/05/2020 06:01:49.537 PM -- hello world\r\n12/05/2020 06:01:49.536 PM -- hello world\r\n12/05/2020 06:01:49.535 PM -- hello world\r\n12/05/2020 06:01:49.535 PM -- hello world\r\n12/05/2020 06:01:49.534 PM -- hello world\r\n12/05/2020 06:01:49.533 PM -- hello world\r\n12/05/2020 06:01:49.532 PM -- hello world\r\n12/05/2020 06:01:49.532 PM -- hello world\r\n12/05/2020 06:01:49.531 PM -- hello world\r\n12/05/2020 06:01:49.530 PM -- hello world\r\n12/05/2020 06:01:49.529 PM -- hello world\r\n12/05/2020 06:01:49.528 PM -- hello world\r\n12/05/2020 06:01:49.528 PM -- hello world\r\n12/05/2020 06:01:49.527 PM -- hello world\r\n12/05/2020 06:01:49.524 PM -- hello world\r\n12/05/2020 06:01:49.523 PM -- hello world\r\n12/05/2020 06:01:49.523 PM -- hello world\r\n12/05/2020 06:01:49.522 PM -- hello world\r\n12/05/2020 06:01:49.521 PM -- hello world\r\n12/05/2020 06:01:49.520 PM -- hello world\r\n12/05/2020 06:01:49.519 PM -- hello world\r\n12/05/2020 06:01:49.518 PM -- hello world\r\n12/05/2020 06:01:49.517 PM -- hello world\r\n12/05/2020 06:01:49.517 PM -- hello world\r\n12/05/2020 06:01:49.516 PM -- hello world\r\n12/05/2020 06:01:49.515 PM -- hello world\r\n12/05/2020 06:01:49.514 PM -- hello world\r\n12/05/2020 06:01:49.513 PM -- hello world\r\n12/05/2020 06:01:49.513 PM -- hello world\r\n12/05/2020 06:01:49.512 PM -- hello world\r\n12/05/2020 06:01:49.511 PM -- hello world\r\n12/05/2020 06:01:49.509 PM -- hello world\r\n12/05/2020 06:01:49.508 PM -- hello world\r\n12/05/2020 06:01:49.507 PM -- hello world\r\n12/05/2020 06:01:49.507 PM -- hello world\r\n12/05/2020 06:01:49.507 PM -- hello world\r\n12/05/2020 06:01:49.506 PM -- hello world\r\n12/05/2020 06:01:49.505 PM -- hello world\r\n12/05/2020 06:01:49.505 PM -- hello world\r\n12/05/2020 06:01:49.504 PM -- hello world\r\n12/05/2020 06:01:49.503 PM -- hello world\r\n12/05/2020 06:01:49.502 PM -- hello world\r\n12/05/2020 06:01:49.499 PM -- hello world\r\n12/05/2020 06:01:49.498 PM -- hello world\r\n12/05/2020 06:01:49.497 PM -- hello world\r\n12/05/2020 06:01:49.496 PM -- hello world\r\n12/05/2020 06:01:49.495 PM -- hello world\r\n12/05/2020 06:01:49.495 PM -- hello world\r\n12/05/2020 06:01:49.494 PM -- hello world\r\n12/05/2020 06:01:49.493 PM -- hello world\r\n12/05/2020 06:01:49.492 PM -- hello world\r\n12/05/2020 06:01:49.491 PM -- hello world\r\n12/05/2020 06:01:49.491 PM -- hello world\r\n12/05/2020 06:01:49.490 PM -- hello world\r\n12/05/2020 06:01:49.489 PM -- hello world\r\n12/05/2020 06:01:49.488 PM -- hello world\r\n12/05/2020 06:01:49.488 PM -- hello world\r\n12/05/2020 06:01:49.487 PM -- hello world\r\n12/05/2020 06:01:49.486 PM -- hello world\r\n12/05/2020 06:01:49.486 PM -- hello world\r\n12/05/2020 06:01:49.485 PM -- hello world\r\n12/05/2020 06:01:49.484 PM -- hello world\r\n12/05/2020 06:01:49.483 PM -- hello world\r\n12/05/2020 06:01:49.483 PM -- hello world\r\n12/05/2020 06:01:49.482 PM -- hello world\r\n12/05/2020 06:01:49.481 PM -- hello world\r\n12/05/2020 06:01:49.477 PM -- hello world\r\n12/05/2020 06:01:49.477 PM -- hello world\r\n12/05/2020 06:01:49.476 PM -- hello world\r\n12/05/2020 06:01:49.475 PM -- hello world\r\n12/05/2020 06:01:49.474 PM -- hello world\r\n12/05/2020 06:01:49.474 PM -- hello world\r\n12/05/2020 06:01:49.473 PM -- hello world\r\n12/05/2020 06:01:49.472 PM -- hello world\r\n12/05/2020 06:01:49.471 PM -- hello world\r\n12/05/2020 06:01:49.471 PM -- hello world\r\n12/05/2020 06:01:49.470 PM -- hello world\r\n12/05/2020 06:01:49.469 PM -- hello world\r\n12/05/2020 06:01:49.468 PM -- hello world\r\n12/05/2020 06:01:49.468 PM -- hello world\r\n12/05/2020 06:01:49.467 PM -- hello world\r\n12/05/2020 06:01:49.466 PM -- hello world\r\n12/05/2020 06:01:49.465 PM -- hello world\r\n12/05/2020 06:01:49.465 PM -- hello world\r\n12/05/2020 06:01:49.464 PM -- hello world\r\n12/05/2020 06:01:49.462 PM -- hello world\r\n12/05/2020 06:01:49.461 PM -- hello world\r\n12/05/2020 06:01:49.460 PM -- hello world\r\n12/05/2020 06:01:49.460 PM -- hello world\r\n12/05/2020 06:01:49.459 PM -- hello world\r\n12/05/2020 06:01:49.458 PM -- hello world\r\n12/05/2020 06:01:49.457 PM -- hello world\r\n12/05/2020 06:01:49.457 PM -- hello world\r\n12/05/2020 06:01:49.456 PM -- hello world\r\n12/05/2020 06:01:49.455 PM -- hello world\r\n12/05/2020 06:01:49.455 PM -- hello world\r\n12/05/2020 06:01:49.454 PM -- hello world\r\n12/05/2020 06:01:49.453 PM -- hello world\r\n12/05/2020 06:01:49.452 PM -- hello world\r\n12/05/2020 06:01:49.451 PM -- hello world\r\n12/05/2020 06:01:49.451 PM -- hello world\r\n12/05/2020 06:01:49.450 PM -- hello world\r\n12/05/2020 06:01:49.449 PM -- hello world\r\n12/05/2020 06:01:49.445 PM -- hello world\r\n12/05/2020 06:01:49.445 PM -- hello world\r\n12/05/2020 06:01:49.444 PM -- hello world\r\n12/05/2020 06:01:49.443 PM -- hello world\r\n12/05/2020 06:01:49.442 PM -- hello world\r\n12/05/2020 06:01:49.442 PM -- hello world\r\n12/05/2020 06:01:49.441 PM -- hello world\r\n12/05/2020 06:01:49.439 PM -- hello world\r\n12/05/2020 06:01:49.439 PM -- hello world\r\n12/05/2020 06:01:49.438 PM -- hello world\r\n12/05/2020 06:01:49.437 PM -- hello world\r\n12/05/2020 06:01:49.437 PM -- hello world\r\n12/05/2020 06:01:49.436 PM -- hello world\r\n12/05/2020 06:01:49.435 PM -- hello world\r\n12/05/2020 06:01:49.433 PM -- hello world\r\n12/05/2020 06:01:49.432 PM -- hello world\r\n12/05/2020 06:01:49.430 PM -- hello world\r\n12/05/2020 06:01:49.429 PM -- hello world\r\n12/05/2020 06:01:49.429 PM -- hello world\r\n12/05/2020 06:01:49.428 PM -- hello world\r\n12/05/2020 06:01:49.427 PM -- hello world\r\n12/05/2020 06:01:49.426 PM -- hello world\r\n12/05/2020 06:01:49.425 PM -- hello world\r\n12/05/2020 06:01:49.425 PM -- hello world\r\n12/05/2020 06:01:49.425 PM -- hello world\r\n12/05/2020 06:01:49.423 PM -- hello world\r\n12/05/2020 06:01:49.423 PM -- hello world\r\n12/05/2020 06:01:49.423 PM -- hello world\r\n12/05/2020 06:01:49.422 PM -- hello world\r\n12/05/2020 06:01:49.420 PM -- hello world\r\n12/05/2020 06:01:49.418 PM -- hello world\r\n12/05/2020 06:01:49.418 PM -- hello world\r\n12/05/2020 06:01:49.417 PM -- hello world\r\n12/05/2020 06:01:49.416 PM -- hello world\r\n12/05/2020 06:01:49.415 PM -- hello world\r\n12/05/2020 06:01:49.413 PM -- hello world\r\n12/05/2020 06:01:49.412 PM -- hello world\r\n12/05/2020 06:01:49.412 PM -- hello world\r\n12/05/2020 06:01:49.411 PM -- hello world\r\n12/05/2020 06:01:49.410 PM -- hello world\r\n12/05/2020 06:01:49.409 PM -- hello world\r\n12/05/2020 06:01:49.409 PM -- hello world\r\n12/05/2020 06:01:49.408 PM -- hello world\r\n12/05/2020 06:01:49.407 PM -- hello world\r\n12/05/2020 06:01:49.406 PM -- hello world\r\n12/05/2020 06:01:49.406 PM -- hello world\r\n12/05/2020 06:01:49.405 PM -- hello world\r\n12/05/2020 06:01:49.396 PM -- hello world\r\n12/05/2020 06:01:49.396 PM -- hello world\r\n12/05/2020 06:01:49.395 PM -- hello world\r\n12/05/2020 06:01:49.395 PM -- hello world\r\n12/05/2020 06:01:49.395 PM -- hello world\r\n12/05/2020 06:01:49.394 PM -- hello world\r\n12/05/2020 06:01:49.394 PM -- hello world\r\n12/05/2020 06:01:49.394 PM -- hello world\r\n12/05/2020 06:01:49.394 PM -- hello world\r\n12/05/2020 06:01:49.393 PM -- hello world\r\n12/05/2020 06:01:49.393 PM -- hello world\r\n12/05/2020 06:01:49.393 PM -- hello world\r\n12/05/2020 06:01:49.392 PM -- hello world\r\n12/05/2020 06:01:49.392 PM -- hello world\r\n12/05/2020 06:01:49.392 PM -- hello world\r\n12/05/2020 06:01:49.392 PM -- hello world\r\n12/05/2020 06:01:49.391 PM -- hello world\r\n12/05/2020 06:01:49.391 PM -- hello world\r\n12/05/2020 06:01:49.391 PM -- hello world\r\n12/05/2020 06:01:49.390 PM -- hello world\r\n12/05/2020 06:01:49.390 PM -- hello world\r\n12/05/2020 06:01:49.390 PM -- hello world\r\n12/05/2020 06:01:49.389 PM -- hello world\r\n12/05/2020 06:01:49.389 PM -- hello world\r\n12/05/2020 06:01:49.389 PM -- hello world\r\n12/05/2020 06:01:49.389 PM -- hello world\r\n12/05/2020 06:01:49.388 PM -- hello world\r\n12/05/2020 06:01:49.388 PM -- hello world\r\n12/05/2020 06:01:49.388 PM -- hello world\r\n12/05/2020 06:01:49.387 PM -- hello world\r\n12/05/2020 06:01:49.386 PM -- hello world\r\n12/05/2020 06:01:49.386 PM -- hello world\r\n12/05/2020 06:01:49.386 PM -- hello world\r\n")   [LabVIEW 2020]
uses:
  Message_Log_Control.ctl
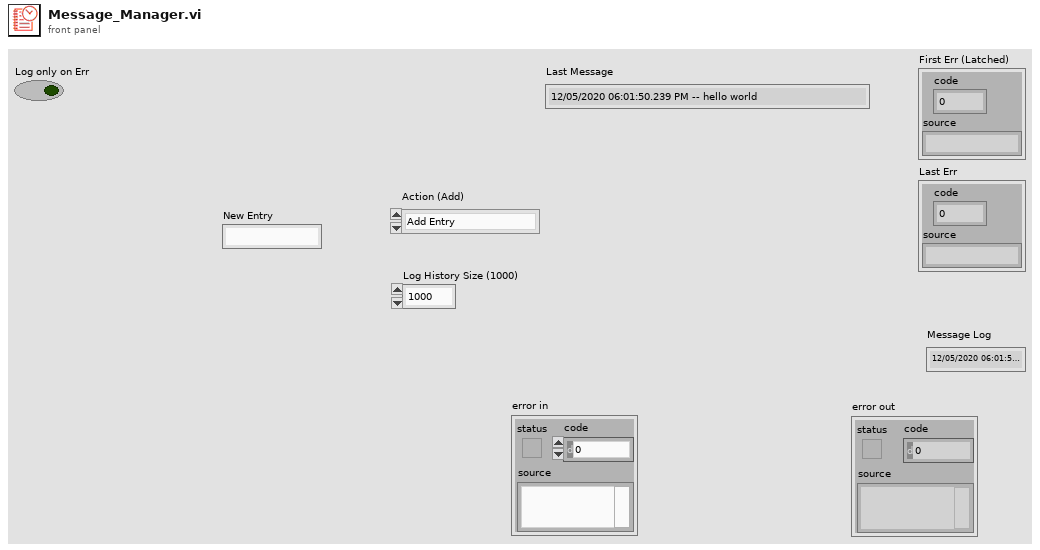
[diagram p1: front panel]
types:
  T1 = typedef "Message_Log_Control.ctl" = enum16{"Add Entry", "Get Log", "Clear Log", "Clear First Error (unlatch)"}
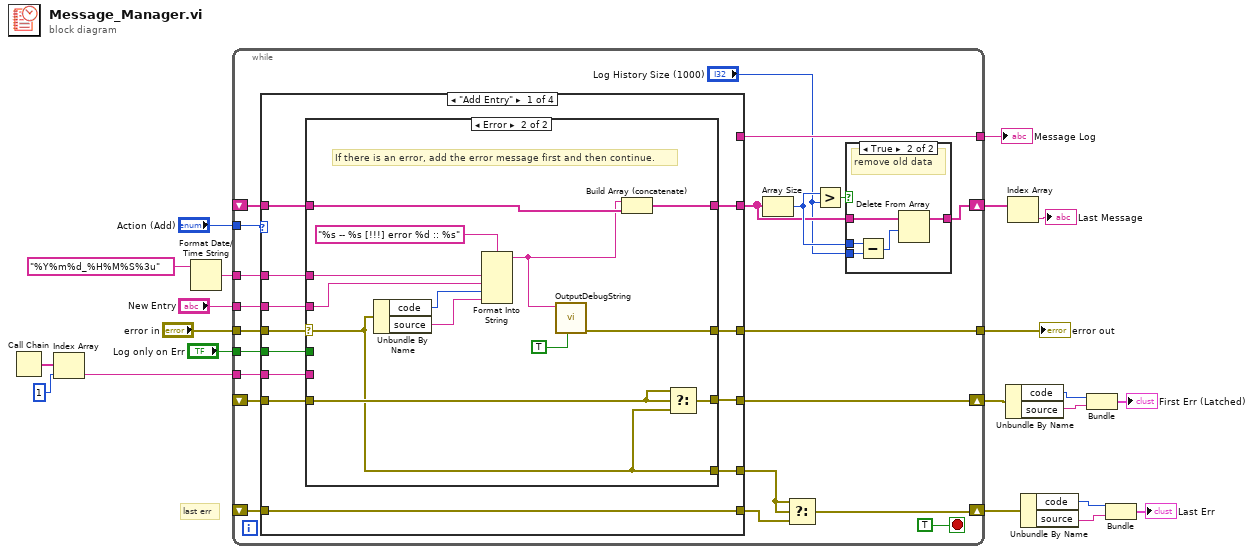
[diagram p0: block diagram]
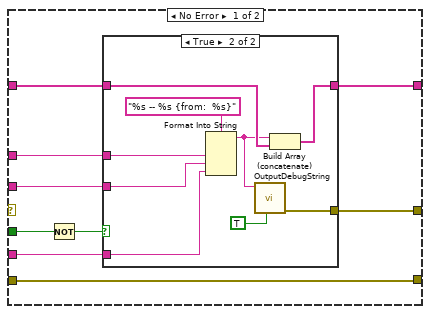
[diagram p3: hidden frame]
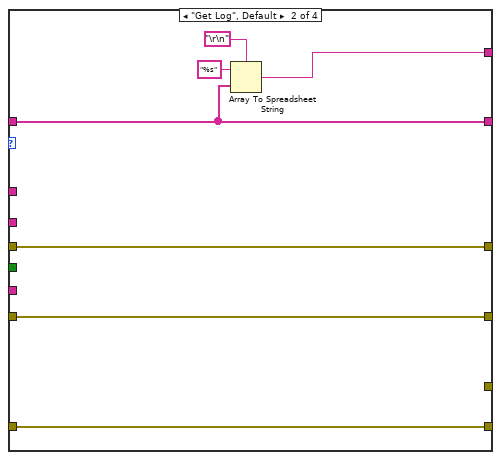
[diagram p5: hidden frame]
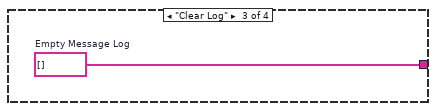
[diagram p6: hidden frame]
diagram:
  # "last err"
  n1 = Call Chain() -> (call chain=w12:string[])
  n2 = Index Array(array=w12, index=1) -> (element=w10:string)
  n3 = Format Date/Time String(time format string (%c)="%Y%m%d_%H%M%S%3u" ("filename time format")) -> (date/time string=w19:string)  [unwired: 2 in]
  n4 = while {
    tunnel: "Action (Add)" -> [w42]
    shift-right: [w32] -> w14
    shift-left: _ -> [w41]
    tunnel: w19 -> [w40]
    tunnel: "New Entry" -> [w39]
    tunnel: [w33] -> w17
    shift-right: [w30] -> w7
    shift-left: _ -> [w29]
    tunnel: w10 -> [w26]
    tunnel: "Log only on Err" -> [w28]
    tunnel: "error in" -> [w38]
    tunnel: [w37] -> w9
    shift-right: [w24] -> w8
    shift-left: _ -> [w22]
    stop <- TRUE stop-if-true
    n5 = case shown="\"Add Entry\"" w42 {
      tunnel: w41 -> [w60 w95 _ w102]
      tunnel: [w59 w95 w100 w102] -> w34
      tunnel: w40 -> [w58 _ _ _]
      tunnel: w39 -> [w57 _ _ _]
      tunnel: w38 -> [w56 w99 _ _]
      tunnel: [w53 w99 _ _] -> w37
      tunnel: [_ w96 _ _] -> w33
      tunnel: [w51 w94 _ _] -> w30
      tunnel: w29 -> [w52 w94 _ _]
      tunnel: w28 -> [w55 _ _ _]
      tunnel: w26 -> [w54 _ _ _]
      tunnel: [w50 _ _ _] -> w25
      tunnel: [w49 w93 _ w101] -> w23
      tunnel: w22 -> [w49 w93 _ w101]
      frame "Add Entry" {
        n6 = case shown="Error" w56 {
          selector: w56 -> [_ w80]
          tunnel: w60 -> [w69 w91]
          tunnel: [w68 w90] -> w59
          tunnel: w58 -> [w67 w92]
          tunnel: w57 -> [w66 w86]
          tunnel: w55 -> [w65 _]
          tunnel: w54 -> [w63 _]
          tunnel: [w61 w81] -> w53
          tunnel: w52 -> [w62 w83]
          tunnel: [w62 w82] -> w51
          tunnel: [_ w80] -> w50
          frame No Error {
            n7 = Not(x=w65) -> (.not. x?=w64:bool)
            n8 = case shown="True" w64 {
              tunnel: [w70 w77] -> w68
              tunnel: w67 -> [_ w78]
              tunnel: w66 -> [_ w75]
              tunnel: w69 -> [w70 w76]
              tunnel: w63 -> [_ w73]
              tunnel: [_ w71] -> w61
              frame False {
                # "nothing to add"
              }
              frame True {
                n9 = Format Into String(format string="%s -- %s {from:  %s}", w78, w75, w73) -> (resulting string=w72:string)  [unwired: 2 in, 1 out]
                n10 = call "OutputDebugString.vi"("Force Log"=TRUE, "log entry string"=w72) -> ("error out"=w71:errorcluster)  [unwired: 6 in, 3 out]
                n11 = Build Array (concatenate)(w72, w76) -> (w77:string[])
              }
            }
          }
          frame Error {
            # "If there is an error, add the error message first and then continue."
            n12 = Unbundle By Name(w80) -> ("code"=w85:i32, "source"=w84:string)
            n13 = Format Into String(format string="%s -- %s [!!!] error %d :: %s", w92, w86, w85, w84) -> (resulting string=w89:string)  [unwired: 2 in, 1 out]
            n14 = call "OutputDebugString.vi"("Force Log"=TRUE, "log entry string"=w89) -> ("error out"=w81:errorcluster)  [unwired: 6 in, 3 out]
            n15 = Build Array (concatenate)(w89, w91) -> (w90:string[])
            n16 = Select(t=w83, s=w83, f=w80) -> (s? t:f=w82:errorcluster)
          }
        }
      }
      frame "Get Log", Default {
        n17 = Array To Spreadsheet String(delimiter (Tab)="\r\n", array=w95, 3:"%s" ("format string")) -> (spreadsheet string=w96:string)
      }
      frame "Clear Log" {
        w100 = string[] []  # Empty Message Log
      }
      frame "Clear First Error (unlatch)" {
      }
    }
    n18 = Array Size(array=w34) -> (size(s)=w35:i32)
    n19 = Select(t=w25, s=w25, f=w23) -> (s? t:f=w24:errorcluster)
    n20 = Greater?(x=w35, y="Log History Size (1000)") -> (0:w36:bool)
    n21 = case shown="True" w36 {
      tunnel: w35 -> [_ w48]
      tunnel: "Log History Size (1000)" -> [_ w47]
      tunnel: [w43 w45] -> w32
      tunnel: w34 -> [w43 w44]
      frame False {
        # "log size is small"
      }
      frame True {
        # "remove old data"
        n22 = Subtract(x=w48, y=w47) -> (x-y=w46:i32)
        n23 = Delete From Array(array=w44, length=w46) -> (array with subset deleted=w45:string[])  [unwired: 1 in, 1 out]
      }
    }
  }
  "error out" <- w9
  "Message Log" <- w17
  n24 = Unbundle By Name(w7) -> ("code"=w6:i32, "source"=w5:string)
  n25 = Index Array(array=w14) -> (element=→"Last Message":string)  [unwired: 1 in]
  n26 = Unbundle By Name(w8) -> ("code"=w2:i32, "source"=w1:string)
  n27 = Bundle("code"=w6, "source"=w5) -> (→"First Err (Latched)":cluster{"code":i32, "source":string})  [unwired: 1 in]
  n28 = Bundle("code"=w2, "source"=w1) -> (→"Last Err":cluster{"code":i32, "source":string})  [unwired: 1 in]
